vi "Byte Buffer.Duplicate.vi"(8 "error in (no error)":errorcluster, 11 "Byte Buffer in":refnum<class "Byte Buffer.lvclass">) -> (0 "error out":errorcluster, 2 "duplicated Byte Buffer":refnum<class "Byte Buffer.lvclass">, 3 "Byte Buffer out":refnum<class "Byte Buffer.lvclass">)   [LabVIEW 2016, in "VeriStand Data.lvlib" / "Byte Buffer.lvclass"]
doc: "Creates a new Byte Buffer instance with the same parameters and data as the provided <B>Byte Buffer</B>."
uses:
  Byte Buffer.lvclass
  Byte Buffer.lvclass/Byte Buffer.ctl
  Memory Management/Memory Management.Handle Return.vi
  VeriStand Data.lvlib
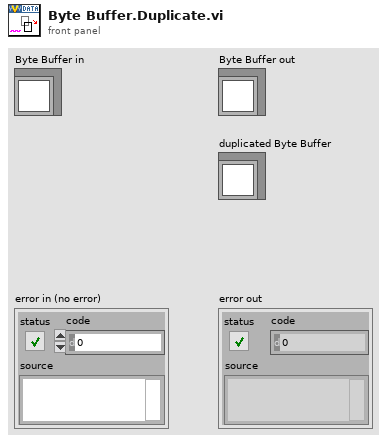
[diagram p1: front panel]
types:
  T1 = enum16{"big-endian, network order", "native, host order", "little-endian"}
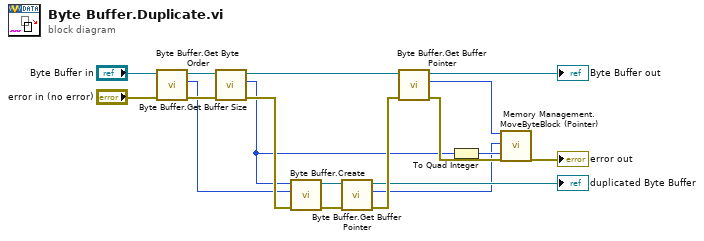
[diagram p0: block diagram]
diagram:
  n1 = call "Byte Buffer.Get Byte Order.vi"("error in (no error)"="error in (no error)", "Byte Buffer in"="Byte Buffer in") -> ("error out"=w14:errorcluster, "byte order"=w13:T1, "Byte Buffer out"=w15:refnum<class "Byte Buffer.lvclass">)  [unwired: 7 in]
  n2 = call "Byte Buffer.Get Buffer Size.vi"("error in (no error)"=w14, "Byte Buffer in"=w15) -> ("error out"=w17:errorcluster, "buffer size"=w6:u64, "Byte Buffer out"=w11:refnum<class "Byte Buffer.lvclass">)  [unwired: 7 in]
  n3 = call "Byte Buffer.Create.vi"("error in (no error)"=w17, "byte order (big-endian)"=w13, "size"=w6) -> ("error out"=w10:errorcluster, "Byte Buffer"=w9:refnum<class "Byte Buffer.lvclass">)  [unwired: 7 in]
  n4 = call "Byte Buffer.Get Buffer Pointer.vi"("error in (no error)"=w10, "Byte Buffer in"=w9) -> ("error out"=w8:errorcluster, "buffer pointer"=w1:u64, "Byte Buffer out"=→"duplicated Byte Buffer":refnum<class "Byte Buffer.lvclass">)  [unwired: 7 in]
  n5 = call "Byte Buffer.Get Buffer Pointer.vi"("error in (no error)"=w8, "Byte Buffer in"=w11) -> ("error out"=w18:errorcluster, "buffer pointer"=w7:u64, "Byte Buffer out"=→"Byte Buffer out":refnum<class "Byte Buffer.lvclass">)  [unwired: 7 in]
  n6 = To Quad Integer(1:w6) -> (0:w4:i64)
  n7 = call "Memory Management.MoveByteBlock (Pointer).vi"("src ptr in"=w7, "dst ptr in"=w1, "size"=w4, "error in (no error)"=w18) -> ("error out"=→"error out":errorcluster)  [unwired: 10 in, 5 out]
